vi "Remove Section.vi"(7 "Section":string, 8 "error in (no error)":errorcluster, 11 "Ini Path in":path) -> (0 "error out":errorcluster, 1 "Section Found?":bool, 3 "Ini Path out":path)   [LabVIEW 2021, in "Config.lvlib"]
uses:
  Config.lvlib
  TypeDefs/Action.ctl
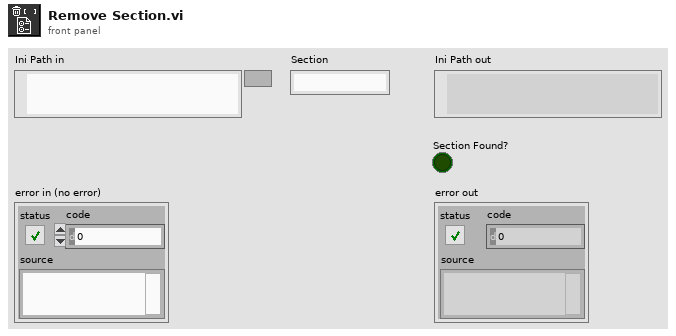
[diagram p1: front panel]
types:
  T1 = typedef "Config.lvlib/Action.ctl" = enum8{"noop", "new", "read_or_create", "read", "write", "remove", "keys", "sections", "remove_section", "import", "export", "get", "set", "pop", "add", "list", "list_sections", "pop_section"}
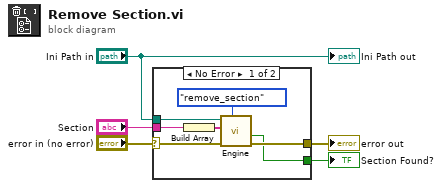
[diagram p0: block diagram]
diagram:
  n1 = case shown="No Error" "error in (no error)" {
    selector: "error in (no error)" -> [w12 w13]
    tunnel: "Ini Path in" -> [w10 _]
    tunnel: [w9 w13] -> w3
    tunnel: "Section" -> [w8 _]
    tunnel: [w6 _] -> w1
    frame No Error {
      n2 = Build Array(w8) -> (w7:string[])
      n3 = call "Engine.vi"("Action"=Action."remove_section", "error in (no error)"=w12, "skvc in"=w7, "INI Path in"=w10) -> ("error out"=w9:errorcluster, "Found?"=w6:bool)  [unwired: 4 in, 2 out]
    }
    frame Error {
    }
  }
  "error out" <- w3
  "Section Found?" <- w1
  "Ini Path out" <- "Ini Path in"
